vi "Modbus Insert Gas State.vi"(10 "Array Input":bool[](array[boolean]), 11 "register values":u16[](array[numeric])) -> (2 "Array Output":bool[](array[boolean]), 3 "FVIR/LDO":bool[](array[boolean]))   [LabVIEW 2020, in "Modbus.lvlib"]
uses:
  Modbus.lvlib
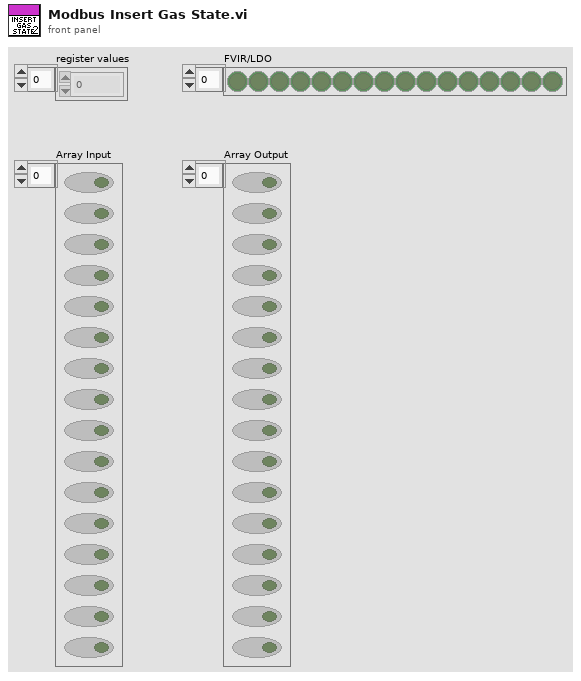
[diagram p1: front panel]
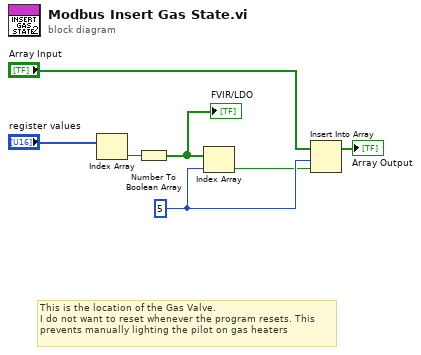
[diagram p0: block diagram]
diagram:
  w7 = 5 ("index")
  # "This is the location of the Gas Valve.\nI do not want to reset whenever the program resets. This\nprevents manually lighting the pilot on gas heaters"
  n1 = Index Array(array="register values") -> (element=w2:u16)  [unwired: 1 in]
  n2 = Number To Boolean Array(number=w2) -> (Boolean array=w3:bool[])
  "FVIR/LDO" <- w3
  n3 = Index Array(array=w3, index=w7) -> (element=w6:bool)
  n4 = Insert Into Array(array="Array Input", index=w7, new element=w6) -> (→"Array Output":bool[])
